vi "EncodeArraySpeedTest.vi"() -> ()   [LabVIEW 2015, in "MsgPack.lvlib"]
uses:
  MsgPack.lvlib
  SubVis/encodeArrayHeader.vi
  EncodeTypes/encodeBaseType.vi
  EncodeTypes/encodeFloat32.vi
panel:
  out "Payload Size":i32
  out "Arrays Match":bool
  out "Speed Improvement":dbl
  out "Auto-Concatenating Array Time":dbl
  out "Preallocate Payload":u8[](array[numeric])
  out "Normal Payload":u8[](array[numeric])
  out "Pre-Allocated Array Time":dbl
  in  "Increment":sgl=3.14 format="%#.20g"
  in  "dimension size":i32=1000
  # "This Example VI is to test the speed difference between different ways to build arrays.\n\nFor Labview 2015, manually Pre-Allocating Arrays is the faster and used through the rest of the MsgPack Library"
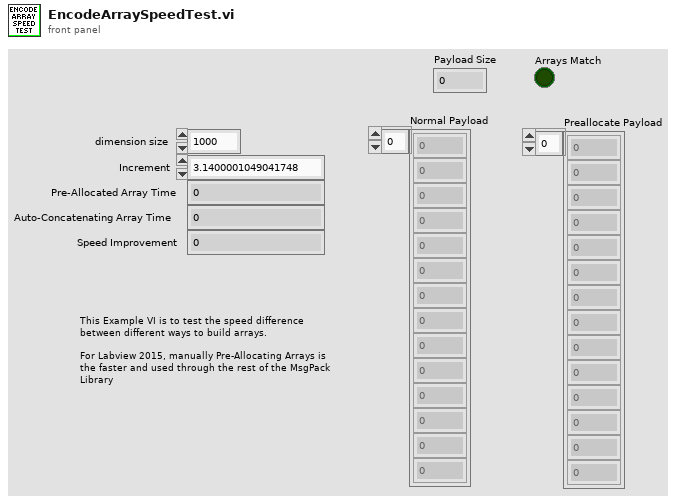
[diagram p1: front panel]
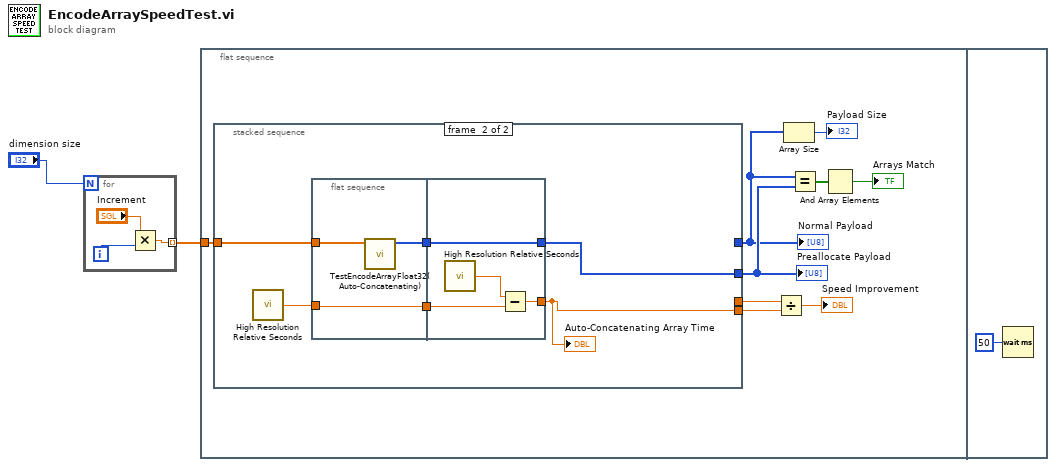
[diagram p0: block diagram]
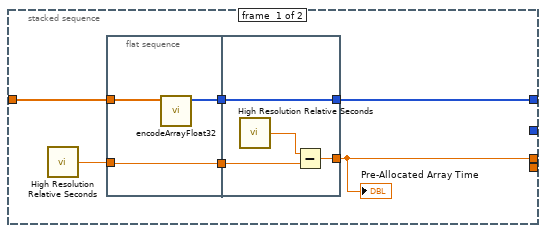
[diagram p2: hidden frame]
diagram:
  n1 = for {
    N: "dimension size" -> [_]
    tunnel: [w3] -> w1 mode=indexing
    i -> [w5]
    n2 = Multiply(x="Increment", y=w5) -> (x*y=w3:sgl)
  }
  n3 = flat-sequence {
    tunnel: w1 -> [w14]
    frame #0 {
      n4 = stacked-sequence {
        tunnel: w14 -> [w20 w33]
        tunnel: [w16 _] -> w13
        tunnel: [_ w29] -> w12
        tunnel: [w15 _] -> w7
        tunnel: [_ w28] -> w10
        frame #0 {
          n5 = call <vilib>:"High Resolution Relative Seconds.vi"() -> ("relative seconds"=w19:dbl)
          n6 = flat-sequence {
            tunnel: w20 -> [w23]
            tunnel: w19 -> [w21]
            tunnel: [w22] -> w18
            tunnel: [w21] -> w17
            tunnel: [w27] -> w15
            tunnel: w18 -> [w27]
            tunnel: w17 -> [w25]
            tunnel: [w24] -> w16
            frame #0 {
              n7 = call "encodeArrayFloat32.vi"("Single Array"=w23) -> ("MessagePack"=w22:u8[])  [unwired: 9 in, 1 out]
            }
            frame #1 {
              n8 = call <vilib>:"High Resolution Relative Seconds.vi"() -> ("relative seconds"=w26:dbl)
              n9 = Subtract(x=w26, y=w25) -> (x-y=w24:dbl)
            }
          }
          "Pre-Allocated Array Time" <- w16
        }
        frame #1 {
          n10 = call <vilib>:"High Resolution Relative Seconds.vi"() -> ("relative seconds"=w32:dbl)
          n11 = flat-sequence {
            tunnel: w33 -> [w35]
            tunnel: w32 -> [w36]
            tunnel: [w34] -> w31
            tunnel: [w36] -> w30
            tunnel: [w40] -> w28
            tunnel: w31 -> [w40]
            tunnel: w30 -> [w38]
            tunnel: [w37] -> w29
            frame #0 {
              n12 = call "TestEncodeArrayFloat32(Auto-Concatenating).vi"("Single Array"=w35) -> ("MessagePack"=w34:u8[])  [unwired: 9 in, 1 out]
            }
            frame #1 {
              n13 = call <vilib>:"High Resolution Relative Seconds.vi"() -> ("relative seconds"=w39:dbl)
              n14 = Subtract(x=w39, y=w38) -> (x-y=w37:dbl)
            }
          }
          "Auto-Concatenating Array Time" <- w29
        }
      }
      "Normal Payload" <- w7
      "Preallocate Payload" <- w10
      n15 = Divide(x=w13, y=w12) -> (x/y=→"Speed Improvement":dbl)
      n16 = Array Size(array=w7) -> (size(s)=→"Payload Size":i32)
      n17 = Equal?(x=w7, y=w10) -> (x = y?=w9:bool[])
      n18 = And Array Elements(Boolean array=w9) -> (logical AND=→"Arrays Match":bool)
    }
    frame #1 {
      n19 = Wait (ms)(milliseconds to wait=u32 50) -> ()  [unwired: 1 out]
    }
  }
